vi "contains.vi"(0 "reference":refnum<class "Graph.lvclass">, 1 "node":refnum<class "AbstractNode.lvclass">, 2 "nodeType(Empty=AllNodeTypesAllaowed)":string[](array[string]), 3 "point2D":T1={"x"=nan, "y"=nan} {"y" format="%.2f"; "x" format="%.2f"}, 5 "error in (no error)":errorcluster, 6 "IgnoreNodes":refnum<class "AbstractNode.lvclass">[](array[class])) -> (14 "reference out":refnum<class "Graph.lvclass">, 15 "contains":bool, 16 "container":refnum<class "AbstractNode.lvclass">, 19 "error out":errorcluster)   [LabVIEW 2012, in "Graph.lvclass"]
doc: "public boolean add(Node n, Point2D p)"
uses:
  <resource>/Framework/Providers/Open_GDS/UML/Graph_class/Graph.lvclass
  <resource>/Framework/Providers/Open_GDS/UML/AbstractNode_class/AbstractNode.lvclass
  <resource>/Framework/Providers/Open_GDS/UML/General/Point/Point Point2D.ctl
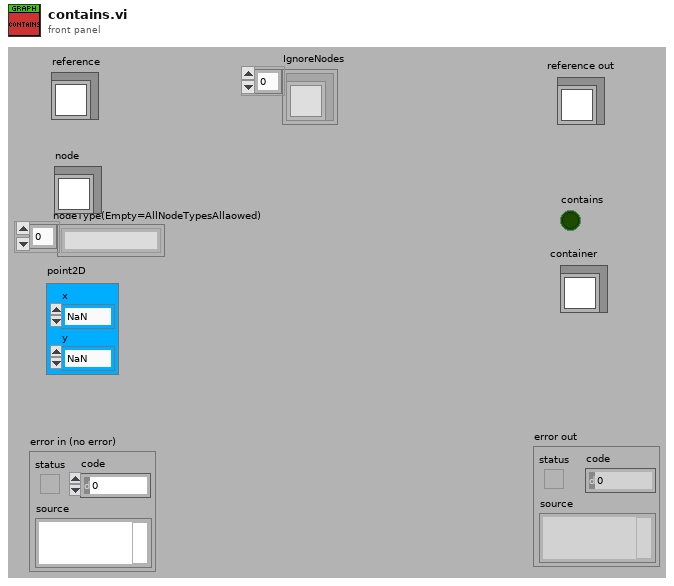
[diagram p1: front panel]
types:
  T1 = typedef "Point Point2D.ctl" = cluster{"x":dbl, "y":dbl}
  T2 = typedef "Graph.lvclass/ObjectAttributes.ctl" = cluster{"nodes":refnum<class "AbstractNode.lvclass">[], "edges":refnum<class "AbstractEdge.lvclass">[], "nodesToBeRemoved":refnum<class "AbstractNode.lvclass">[], "edgesToBeRemoved":refnum<class "AbstractEdge.lvclass">[], "needsLayout":bool, "LayoutNodes":refnum<class "AbstractNode.lvclass">[]}
  T3 = typedef "Rectangle Rectangle2D.ctl" = cluster{"x":dbl, "y":dbl, "width":dbl, "height":dbl}
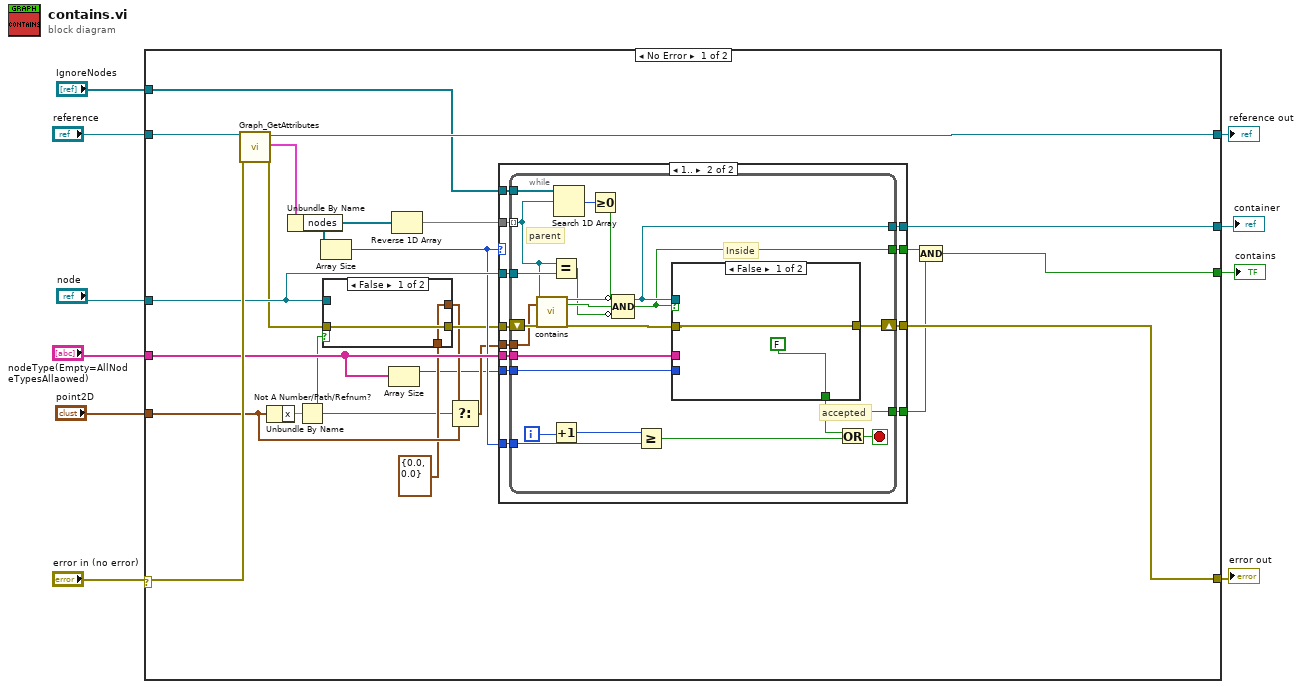
[diagram p0: block diagram]
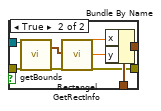
[diagram p2: hidden frame]
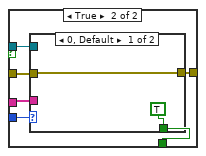
[diagram p4: hidden frame]
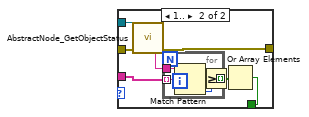
[diagram p5: hidden frame]
diagram:
  n1 = case shown="No Error" "error in (no error)" {
    selector: "error in (no error)" -> [w31 w101]
    tunnel: "reference" -> [w34 w102]
    tunnel: [w33 w101] -> w9
    tunnel: [w32 w102] -> w8
    tunnel: [w30 _] -> w6
    tunnel: "nodeType(Empty=AllNodeTypesAllaowed)" -> [w29 _]
    tunnel: "node" -> [w28 _]
    tunnel: [w27 _] -> w3
    tunnel: "point2D" -> [w26 _]
    tunnel: "IgnoreNodes" -> [w11 _]
    frame No Error {
      n2 = call <resource>:"Graph_GetAttributes.vi"("reference in"=w34, "error in (no error)"=w31) -> ("reference out"=w32:refnum<class "Graph.lvclass">, "Attributes"=w25:T2, "error out"=w19:errorcluster)  [unwired: 15 out]
      n3 = Unbundle By Name(w26) -> ("x"=w16:dbl)
      n4 = Unbundle By Name(w25) -> ("nodes"=w24:refnum<class "AbstractNode.lvclass">[])
      n5 = Not A Number/Path/Refnum?(number/path/refnum=w16) -> (NaN/Path/Refnum?=w13:bool)
      n6 = Array Size(array=w24) -> (size(s)=w21:i32)
      n7 = case shown="False" w13 {
        tunnel: w19 -> [w36 w45]
        tunnel: w28 -> [_ w44]
        tunnel: T1 {"x"=0.0, "y"=0.0} ("point2D") -> [w35 w43]
        tunnel: [w36 w40] -> w17
        tunnel: [w35 w37] -> w15
        frame False {
        }
        frame True {
          n8 = call-dynamic "getBounds.vi"("reference"=w44, "error in (no error)"=w45) -> ("bounds"=w42:T3, "error out"=w41:errorcluster)  [unwired: 16 out]
          n9 = call <resource>:"Rectangel GetRectInfo.vi"("bounds"=w42, "error in (no error)"=w41) -> ("centerX"=w39:dbl, "centerY"=w38:dbl, "error out"=w40:errorcluster)  [unwired: 15 out]
          n10 = Bundle By Name(cluster=w43, "x"=w39, "y"=w38) -> (w37:T1)
        }
      }
      n11 = Array Size(array=w29) -> (size(s)=w12:i32)
      n12 = Reverse 1D Array(array=w24) -> (reversed array=w20:refnum<class "AbstractNode.lvclass">[])
      n13 = Select(t=w15, s=w13, f=w26) -> (s? t:f=w14:T1)
      n14 = case shown="1.." w21 {
        tunnel: w17 -> [w46 w58]
        tunnel: w20 -> [_ w57]
        tunnel: w21 -> [_ w56]
        tunnel: w14 -> [_ w55]
        tunnel: [_ w54] -> w23
        tunnel: [_ w53] -> w22
        tunnel: [w46 w52] -> w33
        tunnel: w29 -> [_ w51]
        tunnel: [_ w50] -> w27
        tunnel: w12 -> [_ w49]
        tunnel: w28 -> [_ w48]
        tunnel: w11 -> [_ w47]
        frame 0, Default {
        }
        frame 1.. {
          n15 = while {
            shift-right: [w71] -> w52
            shift-left: w58 -> [w74]
            tunnel: w57 -> [w59] mode=indexing
            tunnel: w56 -> [w77]
            tunnel: [w65] -> w54
            tunnel: w55 -> [w68]
            tunnel: [w70] -> w53
            tunnel: w51 -> [w69]
            tunnel: [w67] -> w50
            tunnel: w49 -> [w66]
            tunnel: w48 -> [w62]
            tunnel: w47 -> [w63]
            i -> [w79]
            stop <- w75 stop-if-true
            # "parent"
            # "accepted"
            # "Inside"
            n16 = call-dynamic "contains.vi"("reference"=w59, "point2D"=w68, "error in (no error)"=w74) -> ("reference out"=w67:refnum<class "AbstractNode.lvclass">, "contains"=w73:bool, "error out"=w72:errorcluster)  [unwired: 1 in, 13 out]
            n17 = Equal?(x=w59, y=w62) -> (x = y?=w64:bool)
            n18 = Increment(x=w79) -> (x+1=w78:i32)
            n19 = Search 1D Array(1D array=w63, element=w59) -> (index of element=w61:i32)  [unwired: 1 in]
            n20 = Greater Or Equal To 0?(x=w61) -> (x >= 0?=w60:bool)
            n21 = Compound Arithmetic op=AND(invert w60, w73, invert w64) -> (w65:bool)
            n22 = Greater Or Equal?(x=w78, y=w77) -> (x >= y?=w76:bool)
            n23 = case shown="False" w65 {
              tunnel: w72 -> [w81 w87]
              tunnel: w67 -> [_ w86]
              tunnel: [w81 w85] -> w71
              tunnel: [FALSE ("added") w83] -> w70
              tunnel: w69 -> [_ w84]
              tunnel: w66 -> [_ w82]
              frame False {
              }
              frame True {
                n24 = case shown="0, Default" w82 {
                  tunnel: w87 -> [w89 w96]
                  tunnel: w86 -> [_ w95]
                  tunnel: [w89 w94] -> w85
                  tunnel: w84 -> [_ w92]
                  tunnel: [TRUE w90] -> w83
                  frame 0, Default {
                  }
                  frame 1.. {
                    n25 = call <resource>:"AbstractNode_GetObjectStatus.vi"("reference in"=w95, "error in (no error)"=w96) -> ("Class name"=w93:string, "error out"=w94:errorcluster)  [unwired: 16 out]
                    n26 = for {
                      tunnel: [w100] -> w91 mode=indexing
                      tunnel: w93 -> [w98]
                      tunnel: w92 -> [w97] mode=indexing
                      n27 = Match Pattern(string=w98, regular expression=w97) -> (offset past match=w99:i32)  [unwired: 4 out]
                      n28 = Greater Or Equal To 0?(x=w99) -> (x >= 0?=w100:bool)
                    }
                    n29 = Or Array Elements(Boolean array=w91) -> (logical OR=w90:bool)
                  }
                }
              }
            }
            n30 = Or(x=w70, y=w76) -> (x .or. y?=w75:bool)
          }
        }
      }
      n31 = Compound Arithmetic op=AND(w23, w22) -> (w30:bool)
    }
    frame Error {
    }
  }
  "reference out" <- w8
  "error out" <- w9
  "contains" <- w6
  "container" <- w3
